vi "Get DVR.vi"(8 "Error in":errorcluster, 11 "class path":path) -> (0 "Error out":errorcluster, 3 "DVR Out":refnum<data-value>)   [LabVIEW 2020, in "Speed Mode.lvclass"]
uses:
  Speed Mode.lvclass
panel:
  out "Speed Mode out":refnum<class "Speed Mode.lvclass">
  in  "Speed Mode in":refnum<class "Speed Mode.lvclass">
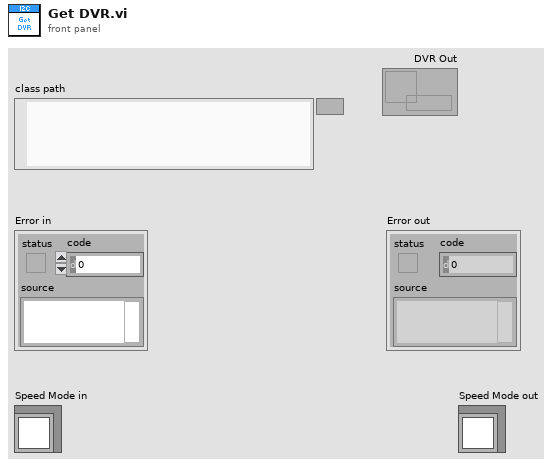
[diagram p1: front panel]
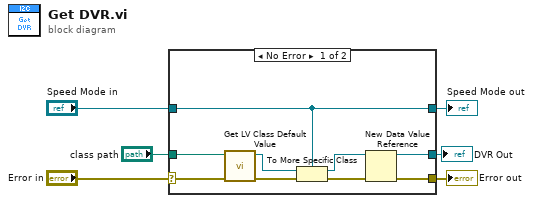
[diagram p0: block diagram]
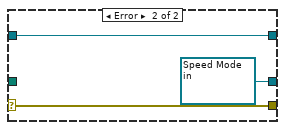
[diagram p2: hidden frame]
diagram:
  n1 = case shown="No Error" "Error in" {
    selector: "Error in" -> [w15 w18]
    tunnel: [w12 w18] -> w5
    tunnel: [w8 w17] -> w3
    tunnel: "Speed Mode in" -> [w8 w17]
    tunnel: "class path" -> [w13 _]
    tunnel: [w11 refnum<data-value> refnum ("data value reference")] -> w1
    frame No Error {
      n2 = call <vilib>:"Get LV Class Default Value.vi"("error in (no error)"=w15, "class path"=w13) -> ("error out"=w14:errorcluster, "object"=w9:refnum<class>)  [unwired: 8 in]
      n3 = To More Specific Class(target class=w8, reference=w9, error in=w14) -> (specific class reference=w7:refnum<class "Speed Mode.lvclass">, error out=w10:errorcluster)
      n4 = New Data Value Reference(data value=w7, error in=w10) -> (data value reference=w11:refnum<data-value>, error out=w12:errorcluster)
    }
    frame Error {
    }
  }
  "Error out" <- w5
  "Speed Mode out" <- w3
  "DVR Out" <- w1
